vi "GetNodeData.vi"(7 "指定从站IP":u32=3232236388 format="%08x", 9 "All RY in":bool[][](array[boolean]), 10 "All RWw in":u16[][](array[numeric]), 11 "从站IP组":u32[](array[numeric])=[3232236289, 3232236388, 4294967295, 4294967295, 4294967295, 3232236290, 4294967295, 3232236291, 4294967295] format="%08x") -> (0 "Node RY":bool[][](array[boolean]), 1 "Node RWw":u16[][](array[numeric]), 3 "占用站数":i32=4)   [LabVIEW 2018]
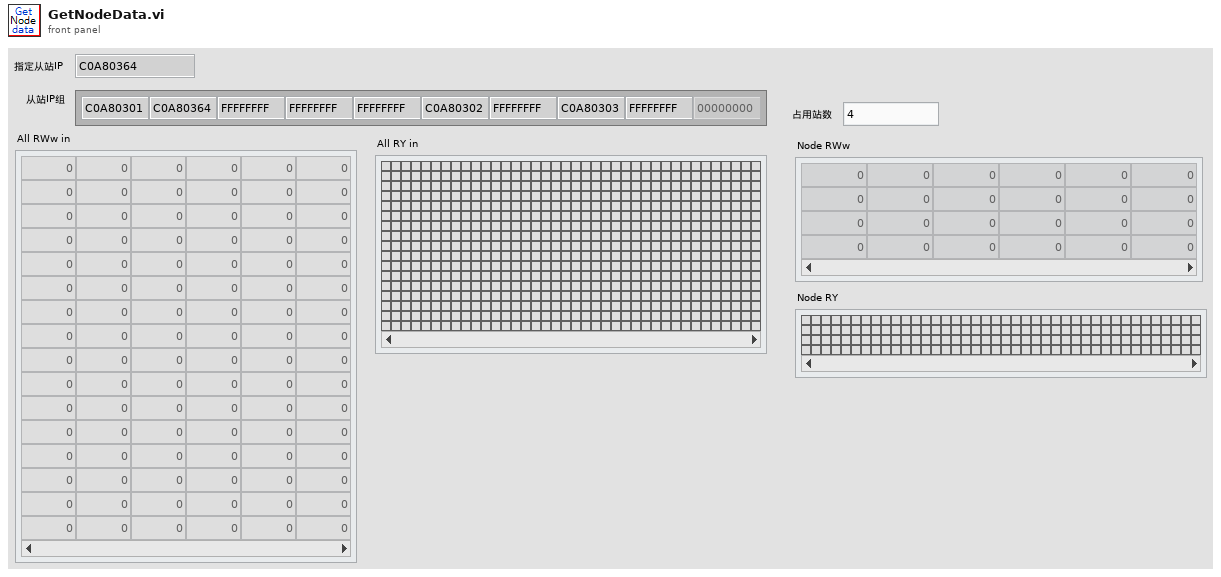
[diagram p1: front panel]
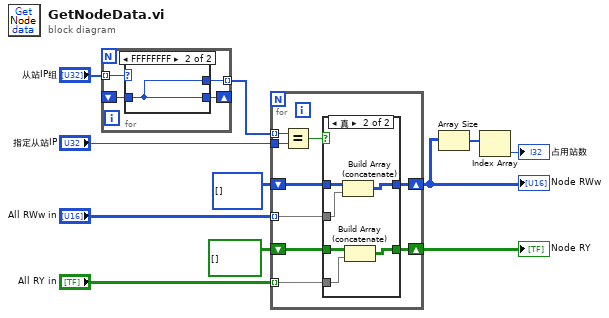
[diagram p0: block diagram]
diagram:
  n1 = for {
    tunnel: "从站IP组" -> [w15] mode=indexing
    shift-right: [w12] -> _
    shift-left: _ -> [w13]
    tunnel: [w14] -> w9 mode=indexing
    n2 = case shown="FFFFFFFF" w15 {
      selector: w15 -> [w16 _]
      tunnel: [w16 w17] -> w14
      tunnel: w13 -> [_ w17]
      tunnel: [w16 w17] -> w12
      frame 0, Default {
      }
      frame -1 {
      }
    }
  }
  n3 = for {
    tunnel: "All RY in" -> [w20] mode=indexing
    tunnel: "All RWw in" -> [w23] mode=indexing
    tunnel: "指定从站IP" -> [w25]
    tunnel: w9 -> [w26] mode=indexing
    shift-right: [w22] -> w5
    shift-left: u16[][] [] -> [w21]
    shift-right: [w18] -> w6
    shift-left: bool[][] [] -> [w19]
    n4 = Equal?(x=w26, y=w25) -> (x = y?=w24:bool)
    n5 = case shown="真" w24 {
      tunnel: w23 -> [_ w34]
      tunnel: [w28 w32] -> w22
      tunnel: w21 -> [w28 w33]
      tunnel: w20 -> [_ w31]
      tunnel: w19 -> [w27 w30]
      tunnel: [w27 w29] -> w18
      frame False {
      }
      frame True {
        n6 = Build Array (concatenate)(w33, w34) -> (w32:u16[][])
        n7 = Build Array (concatenate)(w30, w31) -> (w29:bool[][])
      }
    }
  }
  "Node RWw" <- w5
  "Node RY" <- w6
  n8 = Array Size(array=w5) -> (size(s)=w4:i32[])
  n9 = Index Array(array=w4) -> (element=→"占用站数":i32)  [unwired: 1 in]
